vi "AB_RW_Project_TargetFile_Info.vi"(7 "action":T1, 8 "error in (no error)":errorcluster, 10 "targetfileInfo in":T2, 11 "Object In":T3) -> (0 "error out":errorcluster, 2 "targetfile info":T2, 3 "Object Out":T3)   [LabVIEW 2020]
uses:
  <resource>/Framework/Providers/API/ItemRef.ctl
  <vilib>/AppBuilder/RW_Project/AB_RW_Project_TargetFile_Data.ctl
  <vilib>/AppBuilder/RW_Project/AB_RW_Project_PropBag_Action.ctl
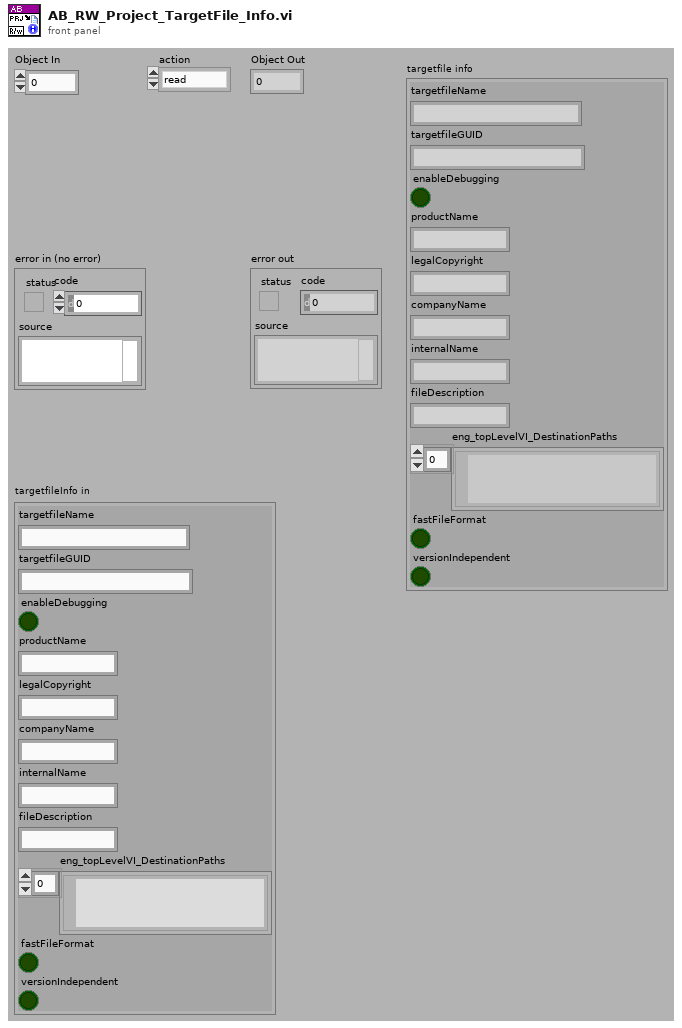
[diagram p1: front panel]
types:
  T1 = typedef "AB_RW_Project_PropBag_Action.ctl" = enum16{"read", "write", "clear", "readPrevious", "writePrevious", "clearPrevious"}
  T2 = typedef "AB_RW_Project_TargetFile_Data.ctl" = cluster{"targetfileName":string, "targetfileGUID":string, "enableDebugging":bool, "productName":string, "legalCopyright":string, "companyName":string, "internalName":string, "fileDescription":string, "eng_topLevelVI_DestinationPaths":path[], "fastFileFormat":bool, "versionIndependent":bool}
  T3 = typedef "ItemRef.ctl" = u64
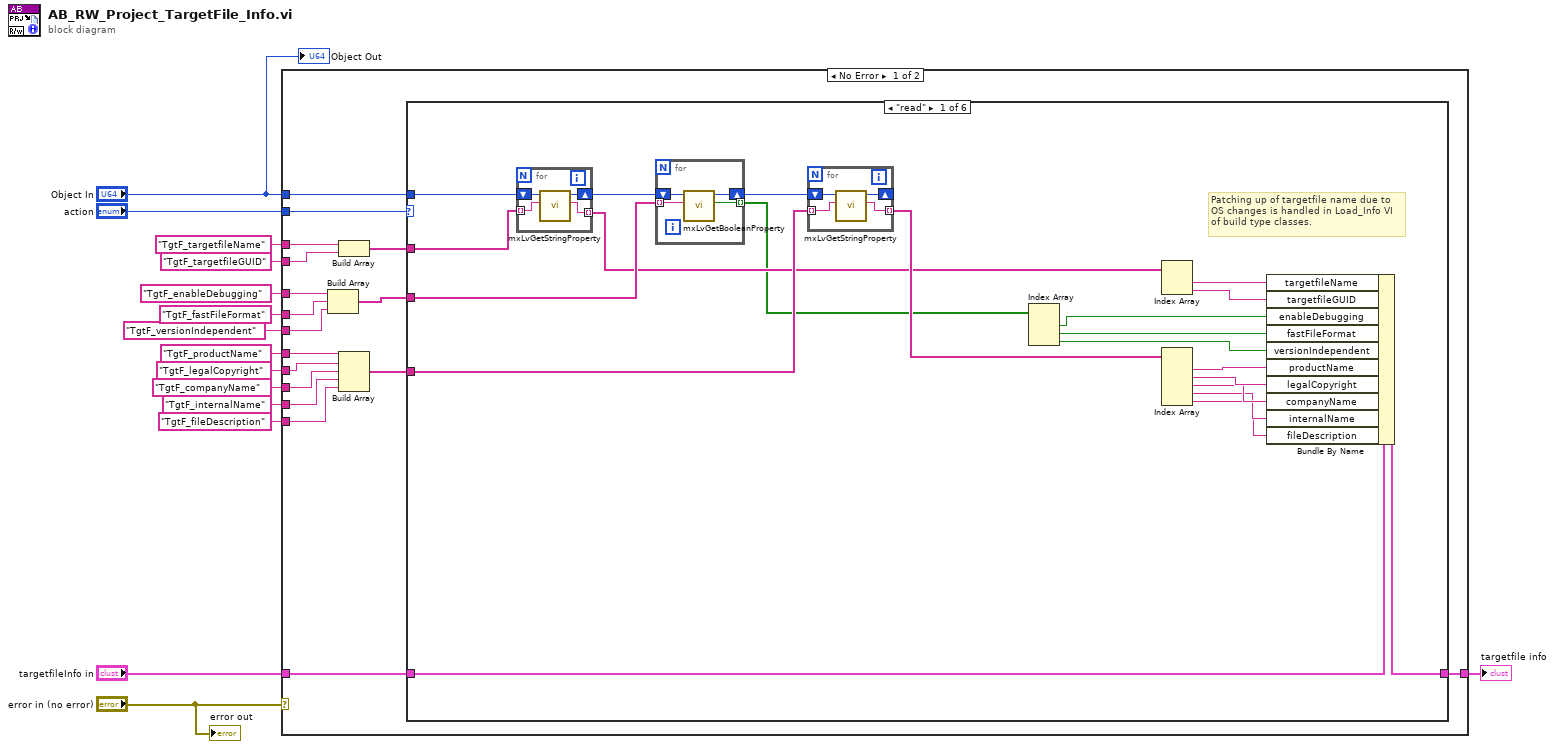
[diagram p0: block diagram]
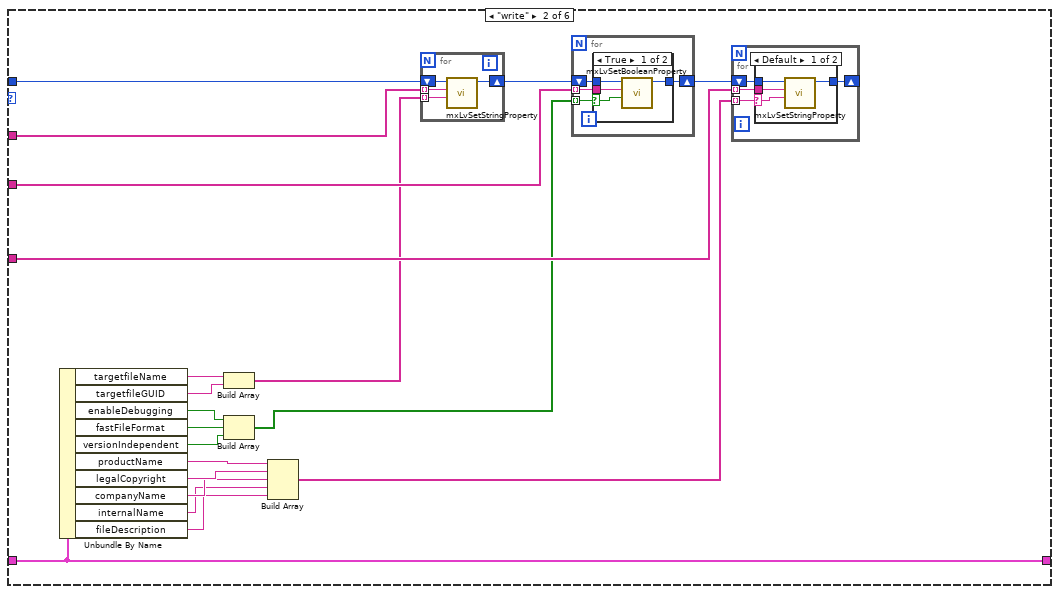
[diagram p2: hidden frame]
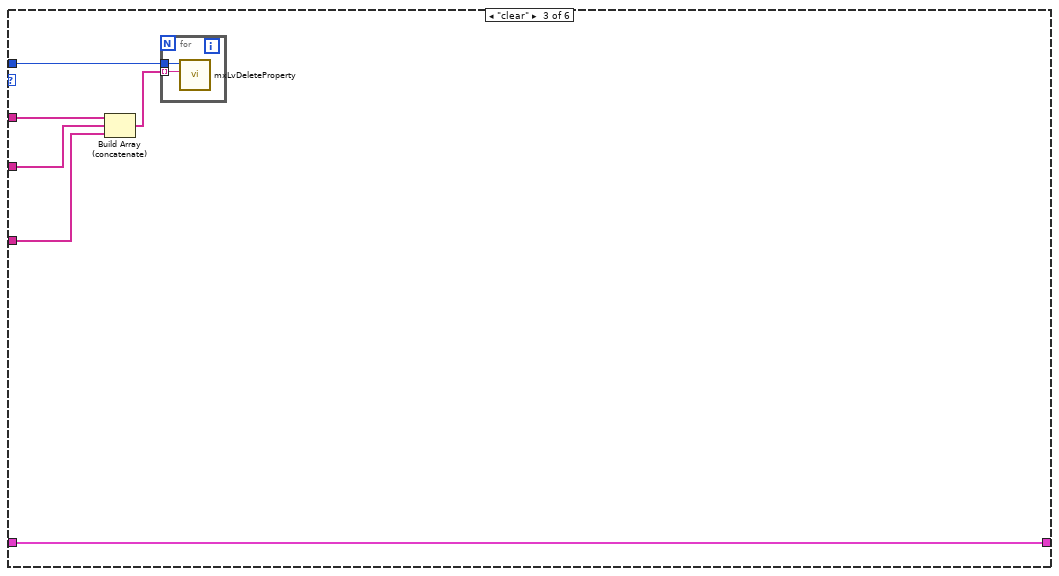
[diagram p5: hidden frame]
diagram:
  n1 = case shown="No Error" "error in (no error)" {
    tunnel: "Object In" -> [w32 _]
    tunnel: [w24 _] -> w13
    tunnel: "targetfileInfo in" -> [w25 _]
    tunnel: "TgtF_targetfileName" ("Tag") -> [w22 _]
    tunnel: "TgtF_enableDebugging" ("Tag") -> [w19 _]
    tunnel: "TgtF_productName" ("Tag") -> [w30 _]
    tunnel: "TgtF_legalCopyright" ("Tag") -> [w31 _]
    tunnel: "TgtF_companyName" ("Tag") -> [w29 _]
    tunnel: "TgtF_internalName" ("Tag") -> [w28 _]
    tunnel: "TgtF_fileDescription" ("Tag") -> [w27 _]
    tunnel: "action" -> [w23 _]
    tunnel: "TgtF_targetfileGUID" ("Tag") -> [w21 _]
    tunnel: "TgtF_fastFileFormat" ("Tag") -> [w17 _]
    tunnel: "TgtF_versionIndependent" ("Tag") -> [w16 _]
    frame No Error {
      n2 = Build Array(w19, w17, w16) -> (w18:string[])
      n3 = Build Array(w22, w21) -> (w20:string[])
      n4 = Build Array(w30, w31, w29, w28, w27) -> (w26:string[])
      n5 = case shown="\"read\"" w23 {
        tunnel: w32 -> [w42 w85 w112 _ _ _]
        tunnel: w18 -> [w52 w83 w111 _ _ _]
        tunnel: w26 -> [w50 w81 w110 _ _ _]
        tunnel: w25 -> [w53 w70 w113 w116 w117 w118]
        tunnel: [w43 w70 w113 w116 w117 w118] -> w24
        tunnel: w20 -> [w41 w74 w108 _ _ _]
        frame "read" {
          # "Patching up of targetfile name due to OS changes is handled in Load_Info VI of build type classes."
          n6 = for {
            shift-right: [w60] -> w37
            shift-left: w42 -> [w61]
            tunnel: w41 -> [w58] mode=indexing
            tunnel: [w59] -> w40 mode=indexing
            n7 = call <resource>:"mxLvGetStringProperty.vi"("Tag"=w58, "Item"=w61) -> ("Value"=w59:string, "Item"=w60:T3)  [unwired: 1 in, 7 out]
          }
          n8 = for {
            tunnel: w52 -> [w57] mode=indexing
            tunnel: [w54] -> w36 mode=indexing
            shift-right: [w56] -> w51
            shift-left: w37 -> [w55]
            n9 = call <resource>:"mxLvGetBooleanProperty.vi"("Tag"=w57, "Item"=w55) -> ("Value"=w54:bool, "Item"=w56:T3)  [unwired: 1 in, 7 out]
          }
          n10 = for {
            shift-right: [w64] -> _
            shift-left: w51 -> [w65]
            tunnel: w50 -> [w62] mode=indexing
            tunnel: [w63] -> w49 mode=indexing
            n11 = call <resource>:"mxLvGetStringProperty.vi"("Tag"=w62, "Item"=w65) -> ("Value"=w63:string, "Item"=w64:T3)  [unwired: 1 in, 7 out]
          }
          n12 = Index Array(array=w36) -> (element #1=w35:bool, element #2=w34:bool, element #3=w33:bool)  [unwired: 3 in]
          n13 = Index Array(array=w40) -> (element #1=w38:string, element #2=w39:string)  [unwired: 2 in]
          n14 = Index Array(array=w49) -> (element #1=w48:string, element #2=w47:string, element #3=w46:string, element #4=w45:string, element #5=w44:string)  [unwired: 5 in]
          n15 = Bundle By Name(cluster=w53, "targetfileName"=w38, "targetfileGUID"=w39, "enableDebugging"=w35, "fastFileFormat"=w34, "versionIndependent"=w33, "productName"=w48, "legalCopyright"=w47, "companyName"=w46, "internalName"=w45, "fileDescription"=w44) -> (w43:T2)
        }
        frame "write" {
          n16 = Unbundle By Name(w70) -> ("targetfileName"=w73:string, "targetfileGUID"=w72:string, "enableDebugging"=w68:bool, "fastFileFormat"=w69:bool, "versionIndependent"=w66:bool, "productName"=w79:string, "legalCopyright"=w80:string, "companyName"=w78:string, "internalName"=w77:string, "fileDescription"=w76:string)
          n17 = Build Array(w73, w72) -> (w71:string[])
          n18 = Build Array(w68, w69, w66) -> (w67:bool[])
          n19 = Build Array(w79, w80, w78, w77, w76) -> (w75:string[])
          n20 = for {
            tunnel: w74 -> [w96] mode=indexing
            tunnel: w71 -> [w95] mode=indexing
            shift-right: [w97] -> w84
            shift-left: w85 -> [w98]
            n21 = call <resource>:"mxLvSetStringProperty.vi"("Value (\"\")"=w95, "Tag"=w96, "Item"=w98) -> ("Item"=w97:T3)  [unwired: 2 in, 6 out]
          }
          n22 = for {
            tunnel: w83 -> [w88] mode=indexing
            tunnel: w67 -> [w86] mode=indexing
            shift-right: [w87] -> w82
            shift-left: w84 -> [w89]
            n23 = case shown="True" w86 {
              selector: w86 -> [w92 _]
              tunnel: w89 -> [w93 w94]
              tunnel: w88 -> [w90 _]
              tunnel: [w91 w94] -> w87
              frame True {
                n24 = call <resource>:"mxLvSetBooleanProperty.vi"("Value (F)"=w92, "Tag"=w90, "Item"=w93) -> ("Item"=w91:T3)  [unwired: 2 in, 6 out]
              }
              frame False {
              }
            }
          }
          n25 = for {
            tunnel: w75 -> [w101] mode=indexing
            shift-right: [w100] -> _
            shift-left: w82 -> [w102]
            tunnel: w81 -> [w99] mode=indexing
            n26 = case shown="Default" w101 {
              selector: w101 -> [w104 _]
              tunnel: w102 -> [w106 w107]
              tunnel: w99 -> [w103 _]
              tunnel: [w105 w107] -> w100
              frame Default {
                n27 = call <resource>:"mxLvSetStringProperty.vi"("Value (\"\")"=w104, "Tag"=w103, "Item"=w106) -> ("Item"=w105:T3)  [unwired: 2 in, 6 out]
              }
              frame "" {
              }
            }
          }
        }
        frame "clear" {
          n28 = Build Array (concatenate)(w108, w111, w110) -> (w109:string[])
          n29 = for {
            tunnel: w112 -> [w115]
            tunnel: w109 -> [w114] mode=indexing
            n30 = call <resource>:"mxLvDeleteProperty.vi"("Tag"=w114, "Item"=w115) -> ()  [unwired: 1 in, 9 out]
          }
        }
        frame "readPrevious" {
        }
        frame "writePrevious" {
        }
        frame "clearPrevious" {
        }
      }
    }
    frame Error {
    }
  }
  "targetfile info" <- w13
  "Object Out" <- "Object In"
  "error out" <- "error in (no error)"
